vi "Global Stop.vi"() -> ()   [LabVIEW 2018]
panel:
  in  "Emergency Stop":bool
  in  "Shutdown":bool
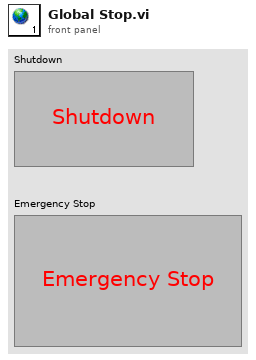
[diagram p1: front panel]
diagram:
